vi "Reset Counters.vi"(8 "error in (no error)":errorcluster, 11 "VISA resource name":refnum<visa-resource-name>) -> (0 "error out":errorcluster, 3 "VISA resource name out":refnum<visa-resource-name>)   [LabVIEW 2011, in "SR400.lvlib"]
doc: "Sending the CR command resets the counters. All\nscanning parameters return to their start values and\npreviously buffered scan data is lost. The CR\ncommand has the same effect as pressing the\nSTOP key twice in succession."
uses:
  SR400.lvlib
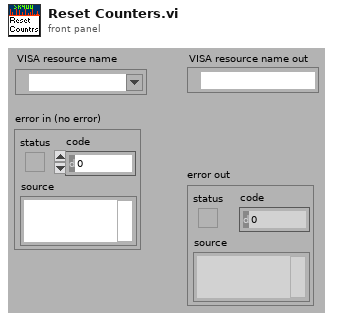
[diagram p1: front panel]
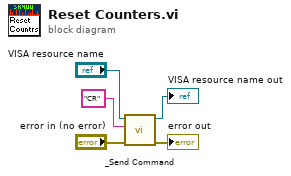
[diagram p0: block diagram]
diagram:
  n1 = call "_Send Command.vi"("error in (no error)"="error in (no error)", "Command"="CR" ("command"), "VISA resource name"="VISA resource name") -> ("error out"=→"error out":errorcluster, "VISA resource name out"=→"VISA resource name out":refnum<visa-resource-name>)  [unwired: 1 in, 6 out]
